vi "Get Theme Data.vi"(8 "error in":errorcluster, 11 "VI Refnum":refnum<vi>) -> (0 "error out":errorcluster, 1 "Theme":u16(ring)=3 items=["Light Theme", "Light Medium Contrast", "Light High Contrast", "Dark Theme", "Dark Medium Contrast", "Dark High Constrast"], 2 "Theme Path":path, 3 "VI Refnum out":refnum<vi>, 4 "Found?":bool)   [LabVIEW 2021, in "TSC Material Theme.lvlib" / "Material Theme.lvclass"]
doc: "Get the VI's user tag data if it exists for the last theme and last theme level applied\n\n<b>Code Developed By:</b>\nDaniel Coons\nTechnology Service Corporation\nwww.tsc.com/atcs"
uses:
  Material Theme.lvclass
  Material Theme.lvclass/Material Theme.ctl
  <vilib>/UserTags/UserTags.lvlib
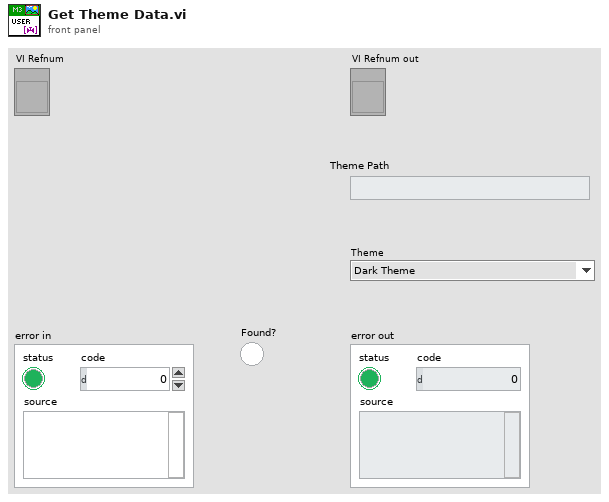
[diagram p1: front panel]
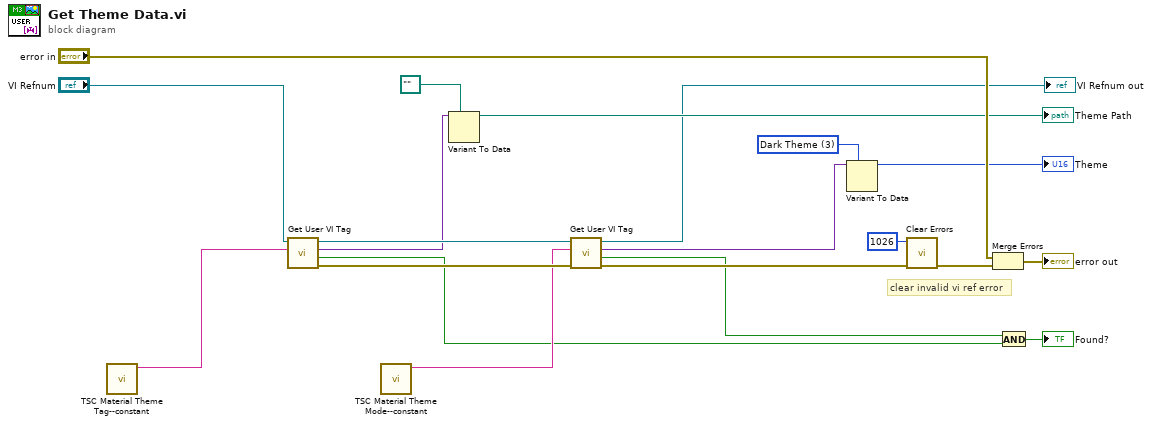
[diagram p0: block diagram]
diagram:
  w7 = u16 3 items=["Light Theme", "Light Medium Contrast", "Light High Contrast", "Dark Theme", "Dark Medium Contrast", "Dark High Constrast"] ("Theme")
  # "clear invalid vi ref error"
  n1 = call "TSC Material Theme Tag--constant.vi"() -> ("Theme Path Tag"=w13:string)  [unwired: 11 in]
  n2 = call <vilib>:"Get User VI Tag.vi"("Tag Name"=w13, "VI Refnum"="VI Refnum") -> ("error out"=w20:errorcluster, "Was Tag Found?"=w4:bool, "Value"=w11:variant, "dup VI Refnum"=w14:refnum<vi>)  [unwired: 6 in]
  n3 = call "TSC Material Theme Mode--constant.vi"() -> ("Theme Path Tag"=w12:string)  [unwired: 11 in]
  n4 = Variant To Data(type=path "", Variant=w11) -> (data=→"Theme Path":path)  [unwired: 1 in, 1 out]
  n5 = call <vilib>:"Get User VI Tag.vi"("error in (no error)"=w20, "Tag Name"=w12, "VI Refnum"=w14) -> ("error out"=w19:errorcluster, "Was Tag Found?"=w3:bool, "Value"=w8:variant, "dup VI Refnum"=→"VI Refnum out":refnum<vi>)  [unwired: 5 in]
  n6 = Variant To Data(type=w7, Variant=w8) -> (data=→"Theme":u16)  [unwired: 1 in, 1 out]
  n7 = call <vilib>:"Clear Errors.vi"("error in (no error)"=w19, "specific error code to clear (0: all)"=1026) -> ("error out"=w16:errorcluster)  [unwired: 4 in, 1 out]
  n8 = Merge Errors("error in", w16) -> (→"error out":errorcluster)
  n9 = And(x=w3, y=w4) -> (x .and. y?=→"Found?":bool)
